vi "ResonanceAnalyzer.vi"() -> ()   [LabVIEW 2014]
uses:
  <vilib>/imath/engines/lvmath2/RunTimeEngine/Managers/WorkSpace/UID Generator.vi
  <vilib>/imath/engines/lvmath2/RunTimeEngine/RangeToken/NIMS_Range.vi
  <instcachedir>/0/NIMS_Range_9BCE657718DF4976A877346C61F22738.lvgen/NIMS_Range_9BCE657718DF4976A877346C61F22738_000.vi
  <vilib>/imath/engines/lvmath2/RunTimeEngine/RunTimeType/NIMS_RunTimeType_From StrictType (excl LVString).vi
  <instcachedir>/0/NIMS_RunTimeType_From StrictType (excl LVString)_15A5391EEA9C4AACB9955AC755B83D29.lvgen/NIMS_RunTimeType_From StrictType (excl LVString)_15A5391EEA9C4AACB9955AC755B83D29_000.vi
  <vilib>/imathl/engines/lvmath/Functions/Error Handling/Create Error.vi
  <vilib>/imath/engines/lvmath2/RunTimeEngine/LocalVariableDefStatement/MC_LocalVariableDefStatement_Display.vi
  <vilib>/imath/engines/lvmath2/RunTimeEngine/ArithmeticOperatorToken/NIMS_ArithmeticOperator_minus.vi
  <instcachedir>/0/NIMS_ArithmeticOperator_minus_39C0593E74DA4138ACA2AB742906488D.lvgen/NIMS_ArithmeticOperator_minus_39C0593E74DA4138ACA2AB742906488D_003.vi
  <vilib>/imath/engines/lvmath2/RunTimeEngine/BuiltInFunctions/randnormal/NIMS_randnormal(1,I32).vi
  <vilib>/imath/engines/lvmath2/RunTimeEngine/ErrorHandling/NIMS_Error From Error Code.vi
  <vilib>/imath/engines/lvmath2/RunTimeEngine/ArithmeticOperatorToken/NIMS_ArithmeticOperator_plus.vi
  <instcachedir>/0/NIMS_ArithmeticOperator_plus_48D6EAACA5D645B09F7EC9C016C2DEA8.lvgen/NIMS_ArithmeticOperator_plus_48D6EAACA5D645B09F7EC9C016C2DEA8_000.vi
  <vilib>/imath/engines/lvmath2/RunTimeEngine/Managers/SymbolTable/Clear UID.vi
  <vilib>/imath/engines/lvmath2/RunTimeEngine/NodeEndStatement/NIMS_NodeEndStatement_Output.vi
  <instcachedir>/0/NIMS_NodeEndStatement_Output_53EC0D466D134D7ABD903AC30B43404B.lvgen/NIMS_NodeEndStatement_Output_53EC0D466D134D7ABD903AC30B43404B_005.vi
  <vilib>/imath/engines/lvmath2/RunTimeEngine/ErrorHandling/NIMS_Finalize Error.vi
  <vilib>/Utility/file.llb/Read From Spreadsheet File (DBL).vi
  <vilib>/imath/engines/lvmath2/RunTimeEngine/Managers/SymbolTable/NIMS_WorkSpace.lvlib
panel:
  out "Cluster":cluster{"Amplitude":dbl, "Q":dbl, "Center":dbl}
  out "XY Graph":cluster{"all rows":dbl[], "Array":dbl[]}[](graph)
  in  "Tab Control":enum32{"Simulation", "Experiment"}(tab)
  in  "Input Parameters":T1
  in  "Data":path
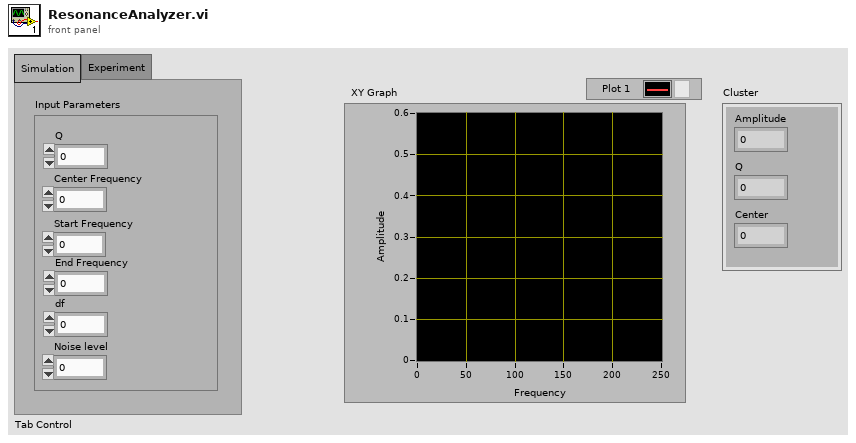
[diagram p1: front panel]
types:
  T1 = cluster{"Q":dbl, "Center Frequency":dbl, "Start Frequency":dbl, "End Frequency":dbl, "df":dbl, "Noise level":dbl}
  T2 = cluster{"Array[0]":dbl, "Array[1]":dbl, "Array[2]":dbl, "Array[3]":dbl, "Array[4]":dbl, "Array[5]":dbl, "Array[6]":dbl, "Array[7]":dbl, "Array[8]":dbl}
  T3 = cluster{"Array[0]":dbl, "Array[1]":dbl, "Array[2]":dbl}
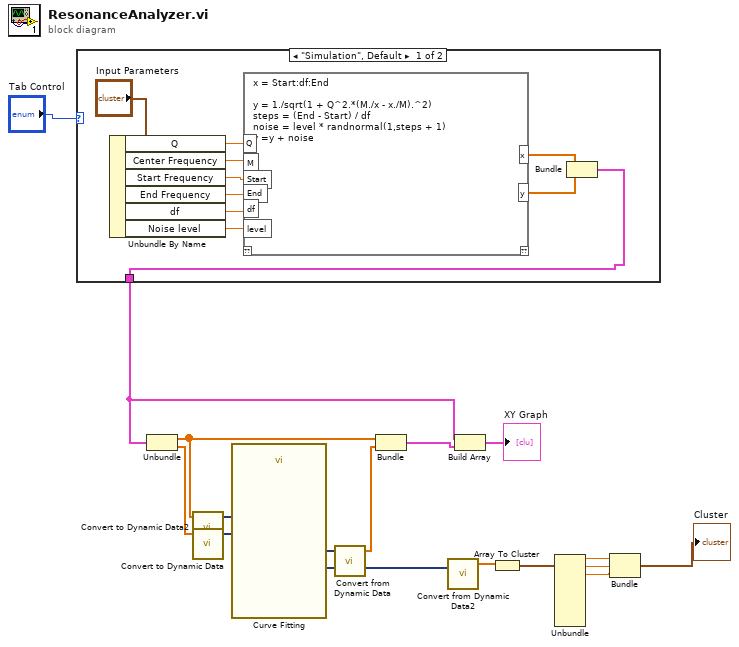
[diagram p0: block diagram]
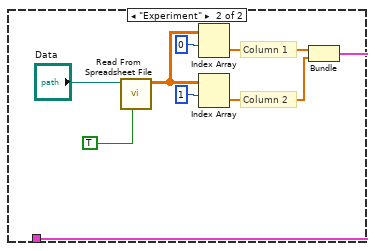
[diagram p2: hidden frame]
diagram:
  n1 = case shown="\"Simulation\", Default" "Tab Control" {
    tunnel: [w18 w199] -> w1
    frame "Simulation", Default {
      n2 = Unbundle By Name("Input Parameters") -> ("Q"=w22:dbl, "Center Frequency"=w23:dbl, "Start Frequency"=w24:dbl, "End Frequency"=w25:dbl, "df"=w26:dbl, "Noise level"=w27:dbl)
      n3 = mathscript code="x = Start:df:End\n\ny = 1./sqrt(1 + Q^2.*(M./x - x./M).^2)\nsteps = (End - Start) / df\nnoise = level * randnormal(1,steps + 1)\ny =y + noise"("Q"=w22, "M"=w23, "Start"=w24, "End"=w25, "df"=w26, "level"=w27) -> ("x"=w21:dbl[], "y"=w19:dbl[])  [unwired: 1 in, 1 out]
      n4 = Bundle("x"=w21, "y"=w19) -> (w18:cluster{"x":dbl[], "y":dbl[]})  [unwired: 1 in]
    }
    frame "Experiment" {
      # "Column 2"
      # "Column 1"
      n5 = call-poly <vilib>:"Read From Spreadsheet File.vi"("transpose (no:F)"=TRUE, "file path (dialog if empty)"="Data") -> ("all rows"=w200:dbl[][])  [unwired: 5 in, 4 out]
      n6 = Index Array(array=w200, index (row)=0) -> (element=w203:dbl[])  [unwired: 1 in]
      n7 = Index Array(array=w200, index (row)=1) -> (element=w204:dbl[])  [unwired: 1 in]
      n8 = Bundle("all rows"=w203, "all rows"=w204) -> (w199:cluster{"all rows":dbl[], "all rows":dbl[]})  [unwired: 1 in]
    }
  }
  n9 = Unbundle(w1) -> ("all rows"=w12:dbl[], "all rows"=w13:dbl[])
  n10 = call "Convert to Dynamic Data2"("Array"=w12) -> ("Dynamic Data Type"=w14:dynamicdata)  [unwired: 3 in]
  n11 = call "Convert to Dynamic Data"("Array"=w13) -> ("Dynamic Data Type"=w15:dynamicdata)  [unwired: 3 in]
  n12 = call "Curve Fitting"("Locations"=w14, "Signals"=w15) -> ("best fit"=w16:dynamicdata, "non-linear coefficients"=w10:dynamicdata)  [unwired: 5 in, 3 out]
  n13 = call "Convert from Dynamic Data"("Dynamic Data Type"=w16) -> ("Array"=w11:dbl[])  [unwired: 3 in]
  n14 = Bundle("all rows"=w12, "Array"=w11) -> (w2:cluster{"all rows":dbl[], "Array":dbl[]})  [unwired: 1 in]
  n15 = call "Convert from Dynamic Data2"("Dynamic Data Type"=w10) -> ("Array"=w9:dbl[])  [unwired: 3 in]
  n16 = Build Array(w1, w2) -> (→"XY Graph":cluster{"all rows":dbl[], "Array":dbl[]}[])
  n17 = Array To Cluster(array=w9) -> (cluster=w8:T2)
  n18 = Unbundle(w8) -> ("Array[0]"=w7:dbl, "Array[1]"=w6:dbl, "Array[2]"=w5:dbl)  [unwired: 6 out]
  n19 = Bundle("Array[0]"=w7, "Array[1]"=w6, "Array[2]"=w5) -> (→"Cluster":T3)  [unwired: 1 in]
